vi "GetImageType.vi"(8 "error in (no error)":errorcluster, 11 "Camera in":refnum<class "CameraI2COUSB.lvclass">) -> (0 "error out":errorcluster, 2 "Image Type":u8 format="%.0x", 3 "Camera out":refnum<class "CameraI2COUSB.lvclass">)   [LabVIEW 2020, in "CameraI2COUSB.lvlib" / "CameraI2COUSB.lvclass"]
uses:
  CameraI2COUSB.lvclass
  CameraI2COUSB.lvclass/CameraI2COUSB.ctl
  Private/TypeDef/RegisterName.ctl
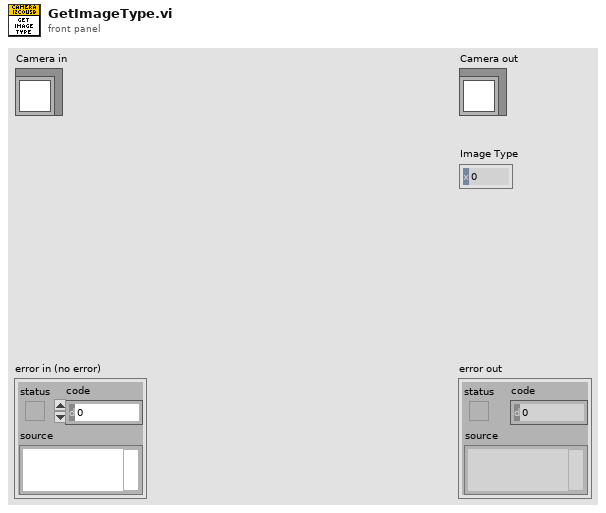
[diagram p1: front panel]
types:
  T1 = typedef "CameraI2COUSB.lvlib/CameraI2COUSB.lvclass/RegisterName.ctl" = enum16{"Clock Rate", "Frame Rate", "Image Type", "Resolution", "Snap", "Start Streaming", "Stop Streaming"}
  T2 = typedef "CameraI2COUSB.lvlib/CameraI2COUSB.lvclass/RegisterInfo.ctl" = cluster{"Address":u16, "Lenght":u32}
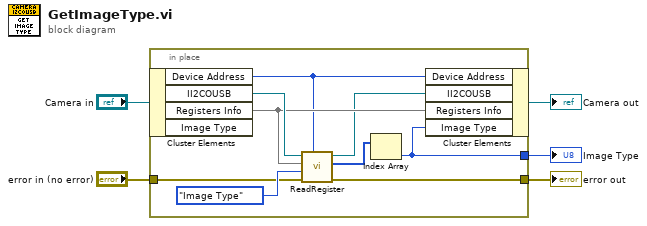
[diagram p0: block diagram]
diagram:
  n1 = in-place {
    in-place-border: "error in (no error)" -> [w10]
    in-place-border: [w9] -> w2
    in-place-border: [w8] -> w1
    n2 = in-place-cluster #1("Camera in") -> ("Device Address"=w11:u8, "II2COUSB"=w14:refnum<class "II2COUSB.lvclass">, "Registers Info"=w13:map{T1, T2})  [unwired: 1 out]
    n3 = call "ReadRegister.vi"("Device Address"=w11, "error in (no error)"=w10, "Register Name"=RegisterName."Image Type", "Registers Info"=w13, "II2COUSB"=w14) -> ("error out"=w9:errorcluster, "DATA"=w7:u8[], "II2COUSB out"=w6:refnum<class "II2COUSB.lvclass">)  [unwired: 4 in]
    n4 = Index Array(array=w7) -> (element=w8:u8)  [unwired: 1 in]
    n5 = in-place-cluster #1("Device Address"=w11, "II2COUSB"=w6, "Registers Info"=w13, "Image Type"=w8) -> (→"Camera out":refnum<class "CameraI2COUSB.lvclass">)
  }
  "error out" <- w2
  "Image Type" <- w1
